vi "Write Single Coil.vi"(8 "error in":errorcluster, 9 "coil value":bool, 10 "address":u16, 11 "device data model in":refnum<class "Standard Data Model.lvclass">) -> (0 "error out":errorcluster, 3 "device data model out":refnum<class "Standard Data Model.lvclass">)   [LabVIEW 2013, in "Modbus Library - Advance.lvlib" / "Standard Data Model.lvclass"]
doc: "Writes the value of a single coil."
uses:
  Standard Data Model.lvclass
  Standard Data Model.lvclass/Standard Data Model.ctl
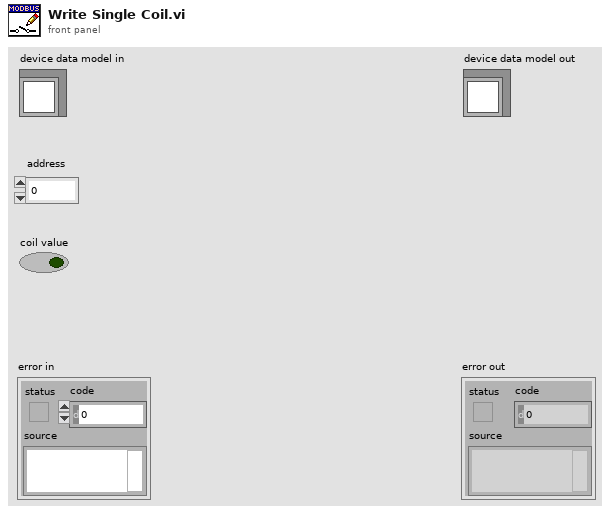
[diagram p1: front panel]
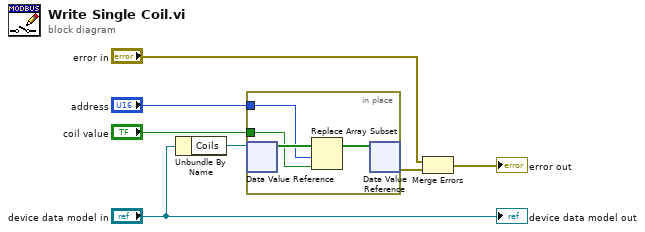
[diagram p0: block diagram]
diagram:
  n1 = Unbundle By Name("device data model in") -> ("Coils"=w6:refnum<data-value>)
  n2 = in-place {
    in-place-border: "coil value" -> [w9]
    in-place-border: "address" -> [w8]
    n3 = in-place-dvr #1(w6) -> (w11:bool[])  [unwired: 1 out]
    n4 = Replace Array Subset(array=w11, new element=w9, index=w8) -> (w10:bool[])
    n5 = in-place-dvr #1(w10) -> (w4:errorcluster)  [unwired: 1 out]
  }
  n6 = Merge Errors("error in", w4) -> (→"error out":errorcluster)
  "device data model out" <- "device data model in"
